vi "SaveToTDMS.vi"(6 "TDMS File Path":path, 8 "error in (no error)":errorcluster, 9 "Label":string, 10 "Task":string, 11 "DAQ_Module in":refnum<class "DAQ_Module.lvclass">) -> (0 "error out":errorcluster, 3 "DAQ_Module out":refnum<class "DAQ_Module.lvclass">)   [LabVIEW 2025, in "DAQ_Module.lvlib" / "DAQ_Module.lvclass"]
uses:
  DAQ_Module.lvclass
  DAQ_Module.lvclass/DAQ_Module.ctl
  DAQ_Abstr/Task_Abstr/Task_Abstr Messages/SaveData Msg/SaveData Msg.lvclass/SaveData Msg.ctl
  <vilib>/ActorFramework/Message Enqueuer/Message Enqueuer.lvclass/Message Enqueuer.ctl
  <vilib>/ActorFramework/Message Enqueuer/Enqueue.vi
  DAQ_Abstr/Task_Abstr/Task_Abstr Messages/SaveData Msg/SaveData Msg.lvclass
  <vilib>/ActorFramework/Message Priority Queue/Priority Enqueue.vi
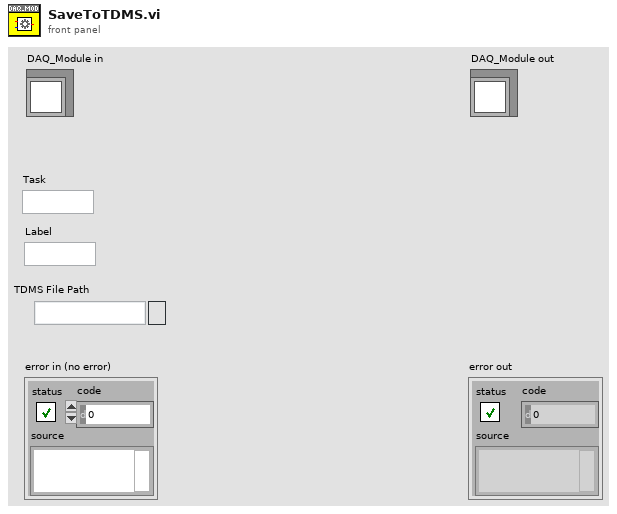
[diagram p1: front panel]
types:
  T1 = map{string, refnum<class "Message Enqueuer.lvclass">}
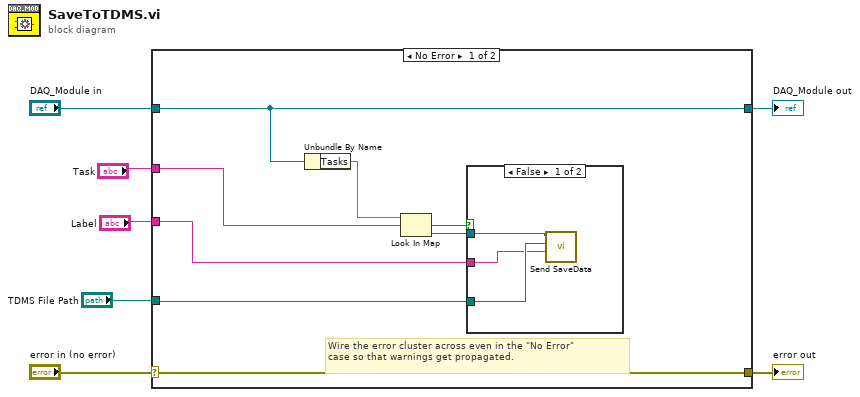
[diagram p0: block diagram]
diagram:
  n1 = case shown="No Error" "error in (no error)" {
    selector: "error in (no error)" -> [w15 w20]
    tunnel: [w15 w20] -> w6
    tunnel: [w11 w19] -> w4
    tunnel: "DAQ_Module in" -> [w11 w19]
    tunnel: "TDMS File Path" -> [w10 _]
    tunnel: "Task" -> [w9 _]
    tunnel: "Label" -> [w8 _]
    frame No Error {
      # "Wire the error cluster across even in the \"No Error\"\ncase so that warnings get propagated."
      n2 = Unbundle By Name(w11) -> ("Tasks"=w14:T1)
      n3 = Look In Map(map=w14, key=w9) -> (key not found?=w12:bool, value=w13:refnum<class "Message Enqueuer.lvclass">)  [unwired: 1 in]
      n4 = case shown="False" w12 {
        tunnel: w13 -> [w18 _]
        tunnel: w8 -> [w16 _]
        tunnel: w10 -> [w17 _]
        frame False {
          n5 = call "Send SaveData.vi"("Label"=w16, "TDMS File Path"=w17, "Message Enqueuer"=w18) -> ()  [unwired: 7 in, 2 out]
        }
        frame True {
        }
      }
    }
    frame Error {
    }
  }
  "error out" <- w6
  "DAQ_Module out" <- w4
